vi "WFS Average Image.vi"(8 "error in (no error)":errorcluster {"code" format="%.0x"}, 10 "Average Count":i32 format="%.0g", 11 "instrument handle":refnum<visa-resource-name>) -> (0 "error out":errorcluster {"code" format="%.0x"}, 2 "Averaged Data Ready":i32, 3 "instrument handle out":refnum<visa-resource-name>)   [LabVIEW 2020]
doc: "This VI generates an averaged image from a number of input camera images in ImageBuf. The VI returns after each call and the summarized image is stored in ImageBufAveraged.\n\nAs soon as the desired number of averages in AverageCount is reached ImageBuf and ImageBufAveraged return both the averaged image data and AverageDataReady returns 1 instead of 0.\n\nNote:\nAs soon as the image size is changed by VI ConfigureCam the averaging process is re-started.\nThis VI is not available in Highspeed Mode!"
uses:
  WFS_32.dll
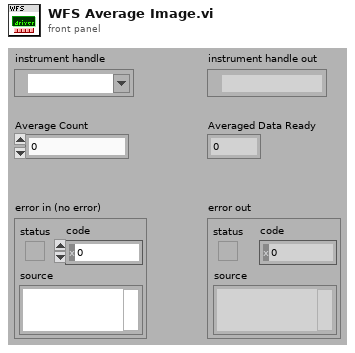
[diagram p1: front panel]
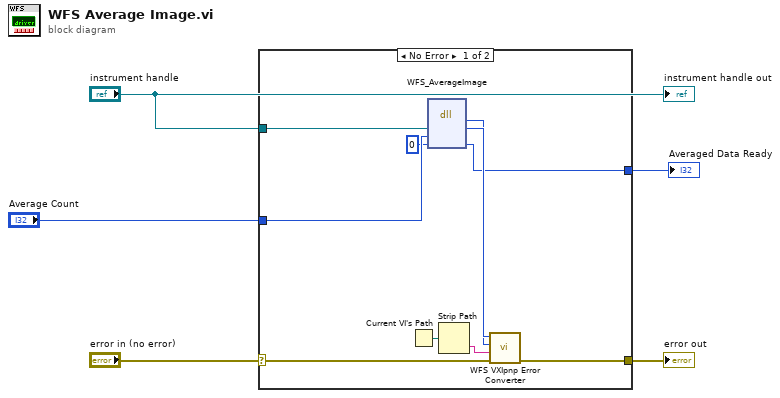
[diagram p0: block diagram]
diagram:
  n1 = case shown="No Error" "error in (no error)" {
    selector: "error in (no error)" -> [w10 w16]
    tunnel: [w9 w16] -> w5
    tunnel: "instrument handle" -> [w14 _]
    tunnel: "Average Count" -> [w8 _]
    tunnel: [w6 _] -> w1
    frame No Error {
      n2 = Current VI's Path() -> (path=w15:path)
      n3 = dll-call lib="WFS_*.*" fn="WFS_AverageImage"("Instrument Handle"=w14, "Average Count"=w8, "Averaged Data Ready"=0) -> (w12:i32, "Instrument Handle"=w13:u32, "Averaged Data Ready"=w6:i32)  [unwired: 4 in, 2 out]
      n4 = Strip Path(path=w15) -> (name=w11:string)  [unwired: 1 out]
      n5 = call "WFS VXIpnp Error Converter.vi"("error in (no error)"=w10, "Name Of VI (\"\")"=w11, "CVI Error Code (0)"=w12, "instrument handle"=w13) -> ("error out"=w9:errorcluster)  [unwired: 6 in, 1 out]
    }
    frame Error {
    }
  }
  "error out" <- w5
  "Averaged Data Ready" <- w1
  "instrument handle out" <- "instrument handle"
